vi "S2C_QuickView.vi"(8 "Error In":errorcluster, 11 "MenuRef":refnum<k9>) -> (0 "Error Out":errorcluster)   [LabVIEW 2015]
doc: "Toggles the \"Local File\" runtime menu item."
uses:
  Globals/S2C_Globals.vi
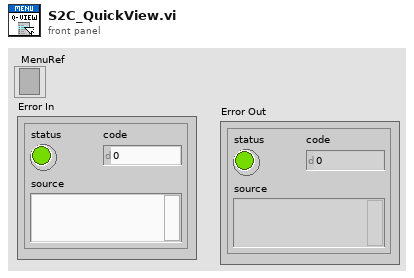
[diagram p1: front panel]
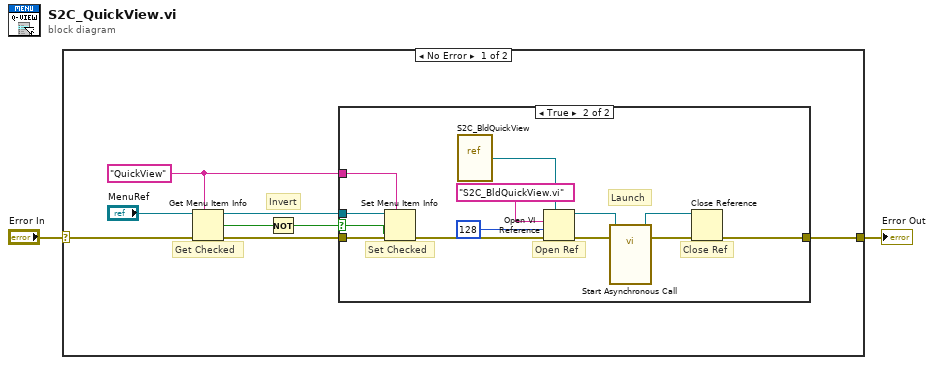
[diagram p0: block diagram]
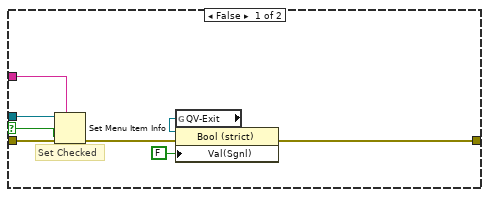
[diagram p2: hidden frame]
diagram:
  n1 = case shown="No Error" "Error In" {
    selector: "Error In" -> [w10 w32]
    tunnel: [w3 w32] -> w1
    frame No Error {
      w8 = "QuickView" ("item tag")
      # "Invert"
      # "Get Checked"
      n2 = Get Menu Item Info(7:w8, 8:w10, 11:"MenuRef") -> (0:w7:errorcluster, 3:w6:refnum<k9>, 4:w5:bool)  [unwired: 4 out]
      n3 = Not(x=w5) -> (.not. x?=w4:bool)
      n4 = case shown="True" w4 {
        selector: w4 -> [w15 w28]
        tunnel: w8 -> [w18 w31]
        tunnel: w7 -> [w17 w30]
        tunnel: w6 -> [w16 w29]
        tunnel: [w13 w21] -> w3
        frame False {
          # "Set Checked"
          n5 = Set Menu Item Info(6:w15, 7:w18, 8:w17, 11:w16) -> (0:w14:errorcluster)  [unwired: 3 in, 1 out]
          n6 = global read "S2C_Globals.vi" "QV-Exit"() -> (w12:refnum<vi>)
          n7 = property class="Bool (strict)"(reference=w12, error in=w14, "Val(Sgnl)"=FALSE ("Value (Signaling)")) -> (error out=w13:errorcluster)  [unwired: 1 out]
        }
        frame True {
          # "Close Ref"
          # "Launch"
          # "Open Ref"
          # "Set Checked"
          n8 = Set Menu Item Info(6:w28, 7:w31, 8:w30, 11:w29) -> (0:w22:errorcluster)  [unwired: 3 in, 1 out]
          n9 = vi-ref "S2C_BldQuickView.vi"() -> (w20:refnum<vi>)
          n10 = Open VI Reference(type specifier VI Refnum (for type only)=w20, vi path="S2C_BldQuickView.vi", options=128, error in (no error)=w22) -> (vi reference=w19:refnum<vi>, error out=w25:errorcluster)  [unwired: 2 in]
          n11 = call-by-ref "Start Asynchronous Call"(reference=w19, error in=w25) -> (reference out=w27:refnum<vi>, error out=w26:errorcluster)  [unwired: 11 in, 1 out]
          n12 = Close Reference(reference=w27, error in (no error)=w26) -> (error out=w21:errorcluster)
        }
      }
    }
    frame Error {
    }
  }
  "Error Out" <- w1
